vi "EXT To SI Noation String.vi"(10 "EXT in":ext format="%.6p") -> (2 "String Out":string)   [LabVIEW 2024]
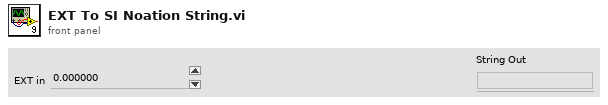
[diagram p1: front panel]
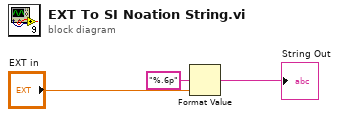
[diagram p0: block diagram]
diagram:
  n1 = Format Value(format string="%.6p", value (0)="EXT in") -> (output string=→"String Out":string)  [unwired: 1 in]
